vi "Initialize Remote Terminals.vi"(8 "error in (no error)":errorcluster, 9 "Next Available Buffer ID in":u16, 10 "Remote Terminals":T1(array[cluster]), 11 "Module Handle in":u32) -> (0 "error out":errorcluster, 1 "Next Available Buffer ID out":u16, 2 "RT Subaddress to Buffer ID Map":T2, 3 "Module Handle out":u32)   [LabVIEW 2020, in "AIM MIL-STD-1553 Engine.lvlib" / "Custom Device.lvlib"]
uses:
  Custom Device.lvlib
  Hardware API/AIM MIL-STD-1553 Hardware API.lvlib
  <instrlib>/_AIM MIL-STD-1553/AIM Controls/1553 Select Direction.ctl
  Implementation/Shared Resources/RT Subaddress to Buffer ID Map.ctl
  Implementation/Shared Resources/Shared Resources.lvclass
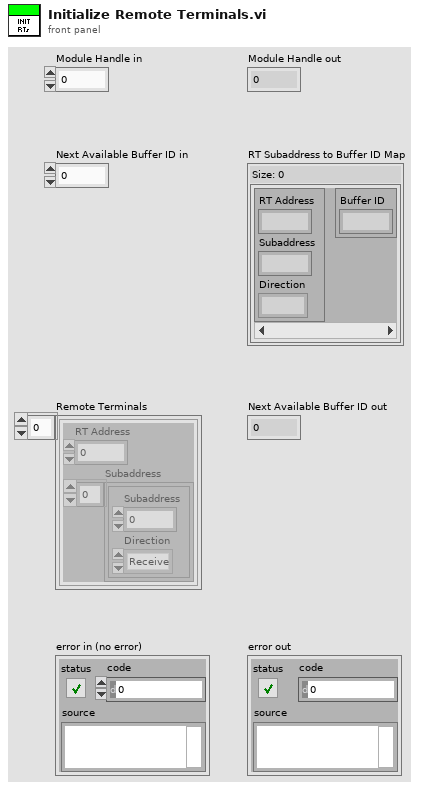
[diagram p1: front panel]
types:
  T1 = cluster{"RT Address":u8, "Subaddress":cluster{"Subaddress":u8, "Direction":enum16{"Receive", "Transmit"}}[]}[]
  T2 = typedef "AIM MIL-STD-1553 Engine.lvlib/Implementation.lvlib/Shared Resources.lvclass/RT Subaddress to Buffer ID Map.ctl" = map{cluster{"RT Address":u8, "Subaddress":u8, "Direction":enum16{"Receive", "Transmit"}}, cluster{"Buffer ID":u16}}
  T3 = typedef "1553 Select Direction.ctl" = enum16{"receive", "transmit"}
  T4 = cluster{"Subaddress":u8, "Direction":enum16{"Receive", "Transmit"}}[]
  T5 = cluster{"RT Address":u8, "Subaddress":u8, "Direction":enum16{"Receive", "Transmit"}}
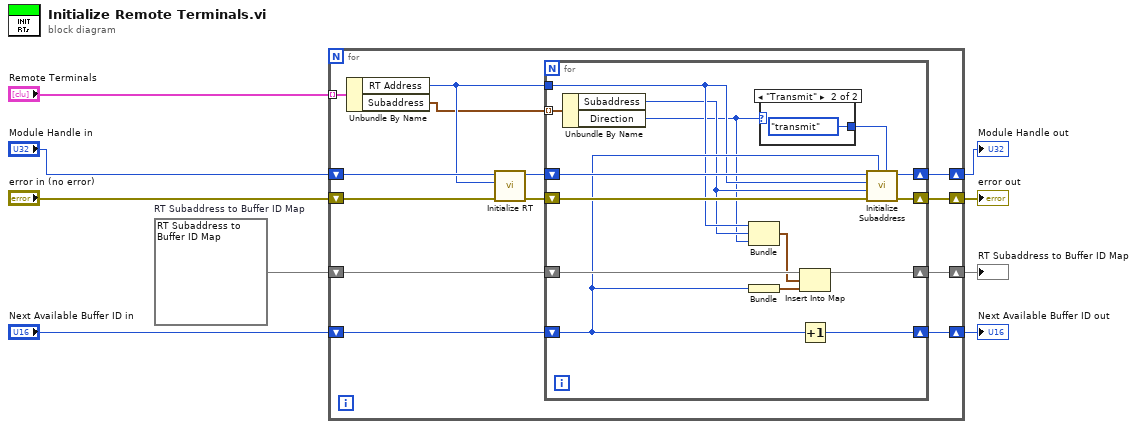
[diagram p0: block diagram]
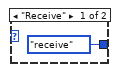
[diagram p2: hidden frame]
diagram:
  w7 = T2 {}  # RT Subaddress to Buffer ID Map
  n1 = for {
    shift-right: [w19] -> w5
    shift-left: "Module Handle in" -> [w22]
    shift-right: [w18] -> w6
    shift-left: "error in (no error)" -> [w21]
    tunnel: "Remote Terminals" -> [w16] mode=indexing
    shift-right: [w12] -> w9
    shift-left: "Next Available Buffer ID in" -> [w13]
    shift-right: [w10] -> w4
    shift-left: w7 -> [w11]
    n2 = Unbundle By Name(w16) -> ("RT Address"=w15:u8, "Subaddress"=w14:T4)
    n3 = call "Initialize RT.vi"("Error In"=w21, "RT Address"=w15, "Module Handle"=w22) -> ("Error Out"=w17:errorcluster, "Module Handle out"=w20:u32)  [unwired: 7 in]
    n4 = for {
      shift-right: [w36] -> w19
      shift-left: w20 -> [w37]
      shift-right: [w34] -> w18
      shift-left: w17 -> [w35]
      tunnel: w15 -> [w27]
      tunnel: w14 -> [w33] mode=indexing
      shift-right: [w31] -> w12
      shift-left: w13 -> [w28]
      shift-right: [w29] -> w10
      shift-left: w11 -> [w30]
      n5 = Unbundle By Name(w33) -> ("Subaddress"=w26:u8, "Direction"=w24:enum16{"Receive", "Transmit"})
      n6 = Bundle("RT Address"=w27, "Subaddress"=w26, "Direction"=w24) -> (w25:T5)  [unwired: 1 in]
      n7 = Bundle("Next Available Buffer ID in"=w28) -> (w23:cluster{"Next Available Buffer ID in":u16})  [unwired: 1 in]
      n8 = case shown="\"Transmit\"" w24 {
        tunnel: [1553_Select_Direction."receive" ("Direction (receive)") 1553_Select_Direction."transmit" ("Direction (receive)")] -> w32
        frame "Receive" {
        }
        frame "Transmit" {
        }
      }
      n9 = Insert Into Map(map in=w30, key=w25, value=w23) -> (map out=w29:T2)  [unwired: 2 out]
      n10 = Increment(x=w28) -> (x+1=w31:u16)
      n11 = call "Initialize Subaddress.vi"("Direction (receive)"=w32, "Buffer Header and Buffer ID"=w28, "Error In"=w35, "Subaddress"=w26, "RT Address"=w27, "Module Handle"=w37) -> ("Error Out"=w34:errorcluster, "Module Handle out"=w36:u32)  [unwired: 4 in]
    }
  }
  "Next Available Buffer ID out" <- w9
  "error out" <- w6
  "Module Handle out" <- w5
  "RT Subaddress to Buffer ID Map" <- w4
